vi "Check if Actuator has Error.vi"(7 "error in (no error)":errorcluster, 9 "Actuator Name":string, 10 "UTP IO Session in":T1) -> (0 "error out":errorcluster, 2 "Actuator has Error?":bool, 3 "UTP IO Session out":T1)   [LabVIEW 2023, in "Actuators.lvlib"]
doc: "Check if Actuator has Error"
uses:
  Actuators.lvlib
  <vilib>/Noffz/UTP IO/UTP IO Library/Typedefs/Session Handle.ctl
  <vilib>/Noffz/UTP IO/UTP IO Library/UTP IO Pool Session.lvclass
  <vilib>/Noffz/UTP IO/UTP IO Library/methods/poly/plc/Read PLC Variable (Boolean).vi
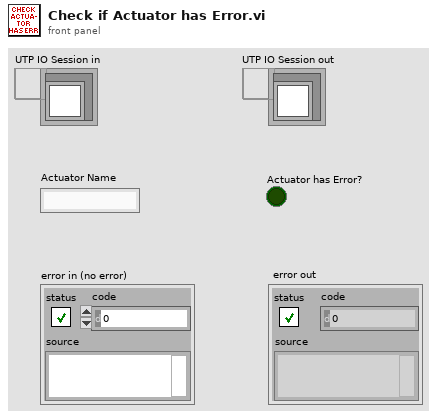
[diagram p1: front panel]
types:
  T1 = typedef "UTP IO Library.lvlib/UTP IO Pool Session.lvclass/Session Handle.ctl" = refnum<data-value>
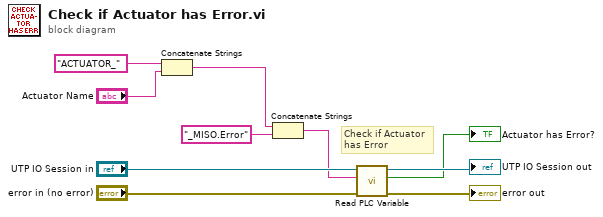
[diagram p0: block diagram]
diagram:
  # "Check if Actuator\nhas Error"
  n1 = Concatenate Strings("ACTUATOR_" ("string"), "Actuator Name") -> (w4:string)
  n2 = Concatenate Strings(w4, "_MISO.Error" ("string")) -> (w9:string)
  n3 = call-poly <vilib>:"Read PLC Variable.vi"("error in (no error)"="error in (no error)", "variable name"=w9, "UTP IO Session in"="UTP IO Session in") -> ("error out"=→"error out":errorcluster, "value"=→"Actuator has Error?":bool, "UTP IO Session out"=→"UTP IO Session out":T1)  [unwired: 6 in]
